vi "tvac_gui_test_mini.vi"() -> ()   [LabVIEW 2017]
panel:
  out "value 2":T1
  out "value":string
  out "JSON string":string
  in  "Tab Control":enum32{"Page 1", "Page 2"}(tab)
  in  "Path":path=path "C:/Users/stefan/Documents/UCryo/TVAC.git/branches/stefanDev/head/LabVIEW/Sandbox/TVAC_GUI/tc_example_1.txt"
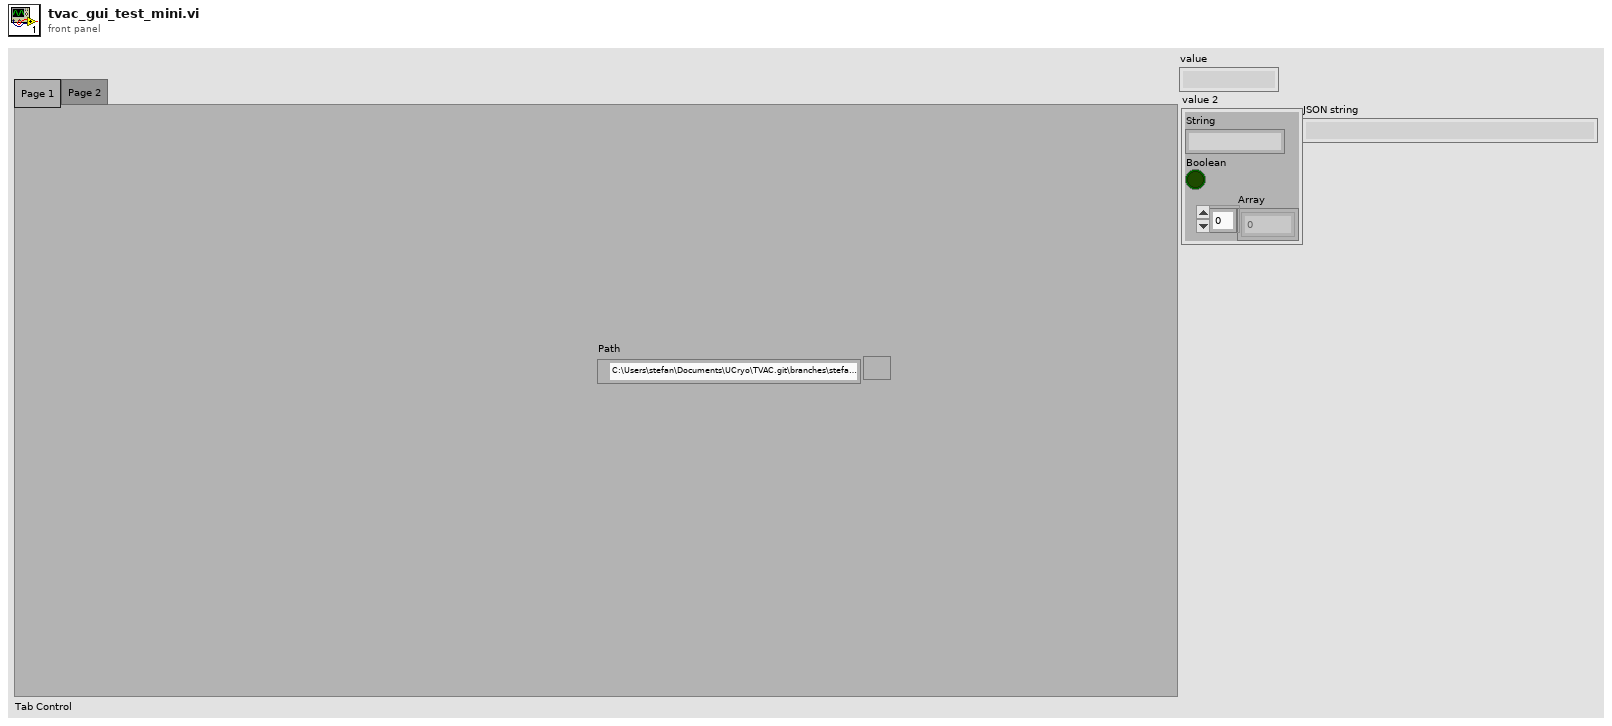
[diagram p1: front panel]
types:
  T1 = cluster{"String":string, "Boolean":bool, "Array":dbl[]}
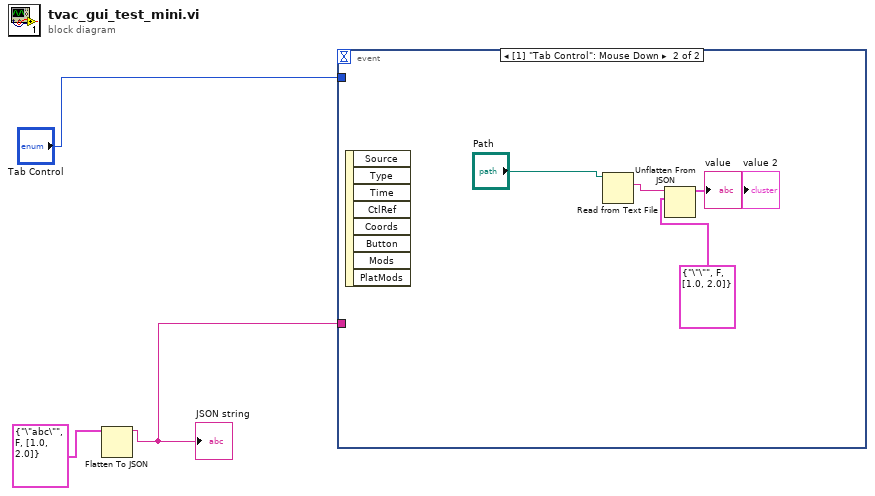
[diagram p0: block diagram]
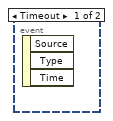
[diagram p2: hidden frame]
diagram:
  n1 = Flatten To JSON(anything=T1 {"String"="\"abc\"", "Boolean"=FALSE, "Array"=[1.0, 2.0]} ("Cluster")) -> (JSON string=w1:string)  [unwired: 2 in, 1 out]
  "JSON string" <- w1
  n2 = event shown="[1] \"Tab Control\": Mouse Down" {
    selector: _ -> [_ _]
    dyn-events: _ -> [_ _]
    timeout: _ -> [_ _]
    tunnel: "Tab Control" -> [_ _]
    tunnel: w1 -> [_ _]
    event Timeout {
      n3 = event-data() -> ()  [unwired: 1 in, 3 out]
    }
    event "Tab Control": Mouse Down {
      n4 = event-data() -> ()  [unwired: 1 in, 8 out]
      n5 = Read from Text File(file (use dialog)="Path") -> (text=w4:string)  [unwired: 3 in, 3 out]
      n6 = Unflatten From JSON(JSON string=w4, type and defaults=T1 {"String"="\"\"", "Boolean"=FALSE, "Array"=[1.0, 2.0]} ("Cluster")) -> (value=→"value 2":T1)  [unwired: 5 in, 1 out]
    }
  }
